vi "ForwardForTime.vi"(8 "error in":errorcluster, 10 "Time (ms)":u32, 11 "Speed/Direction":dbl) -> (0 "error out":errorcluster)   [LabVIEW 2016]
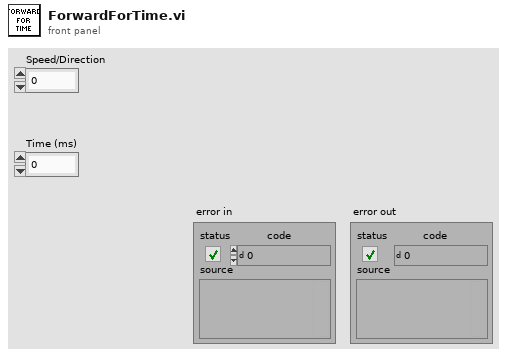
[diagram p1: front panel]
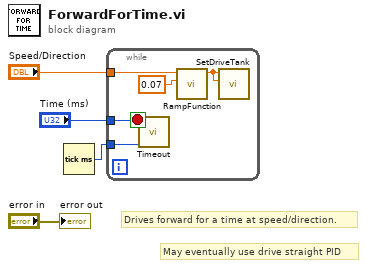
[diagram p0: block diagram]
diagram:
  # "May eventually use drive straight PID"
  # "Drives forward for a time at speed/direction."
  n1 = Tick Count (ms)() -> (millisecond timer value=w2:u32)
  n2 = while {
    tunnel: "Time (ms)" -> [w10]
    tunnel: "Speed/Direction" -> [w6]
    tunnel: w2 -> [w8]
    stop <- w9 stop-if-true
    n3 = call "Timeout.vi"("Start Time In"=w8, "Time Limit"=w10) -> ("Timeout"=w9:bool)  [unwired: 8 in, 1 out]
    n4 = call "RampFunction.vi"("Max Rate"=0.07, "Input"=w6) -> ("Output"=w5:dbl)  [unwired: 9 in]
    n5 = call "SetDriveTank.vi"("Right"=w5, "Left"=w5) -> ()  [unwired: 9 in, 1 out]
  }
  "error out" <- "error in"
